vi "Do.vi"(8 "error in (no error)":errorcluster, 10 "Actor in":refnum<class "Actor.lvclass">, 11 "Mouseover Panel Object Msg":refnum<class "Mouseover Panel Object Msg.lvclass">) -> (0 "error out":errorcluster, 2 "Actor out":refnum<class "Actor.lvclass">)   [LabVIEW 2017, in "Pane Relief Main UI.lvlib" / "Mouseover Panel Object Msg.lvclass"]
doc: "This VI delivers the message to the actor by calling the appropriate method(s) on the actor."
uses:
  Mouseover Panel Object Msg.lvclass
  <vilib>/ActorFramework/Actor/Actor.lvclass
  Pane Relief Main UI/Pane Relief Main UI.lvclass
  C:/Program Files (x86)/National Instruments/LabVIEW 2017/vi.lib/ActorFramework/Actor/Actor.lvclass
  Mouseover Panel Object Msg.lvclass/Mouseover Panel Object Msg.ctl
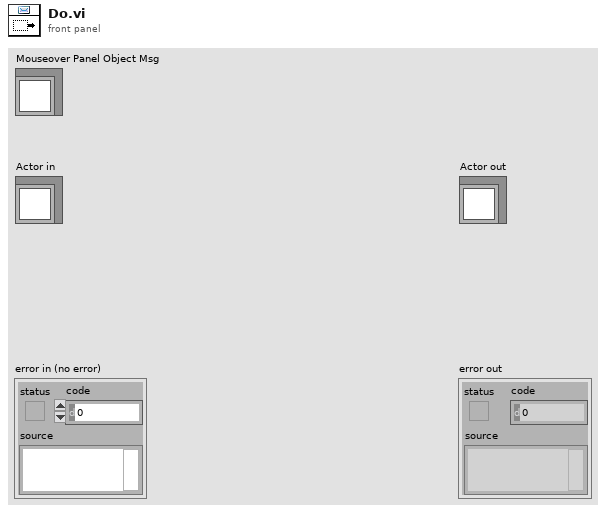
[diagram p1: front panel]
types:
  T1 = typedef "LVPoint32TypeDef.ctl" = cluster{"Horizontal":i32, "Vertical":i32}
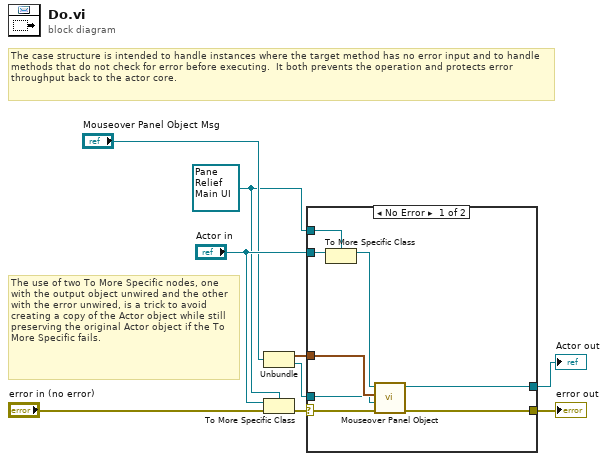
[diagram p0: block diagram]
diagram:
  w4 = refnum<class "Pane Relief Main UI.lvclass"> refnum ("Actor in")
  # "The use of two To More Specific nodes, one with the output object unwired and the other with the error unwired, is a trick to avoid creating a copy of the Actor object while still preserving the original Actor object if the To More Specific fails."
  # "The case structure is intended to handle instances where the target method has no error input and to handle methods that do not check for error before executing.  It both prevents the operation and protects error throughput back to the actor core."
  n1 = Unbundle("Mouseover Panel Object Msg") -> (w2:T1, w1:refnum<k4>)
  n2 = To More Specific Class(target class=w4, reference="Actor in", error in="error in (no error)") -> (error out=w3:errorcluster)  [unwired: 1 out]
  n3 = case shown="No Error" w3 {
    selector: w3 -> [w15 w19]
    tunnel: [w17 w19] -> w9
    tunnel: [w16 w18] -> w8
    tunnel: "Actor in" -> [w14 w18]
    tunnel: w4 -> [w13 _]
    tunnel: w2 -> [w11 _]
    tunnel: w1 -> [w10 _]
    frame No Error {
      n4 = To More Specific Class(target class=w13, reference=w14) -> (specific class reference=w12:refnum<class "Pane Relief Main UI.lvclass">)  [unwired: 1 in, 1 out]
      n5 = call-dynamic "Mouseover Panel Object.vi"("Error In"=w15, "Occurrence"=w10, "Coords"=w11, "Pane Relief Main UI in"=w12) -> ("Error Out"=w17:errorcluster, "Pane Relief Main UI out"=w16:refnum<class "Pane Relief Main UI.lvclass">)  [unwired: 6 in]
    }
    frame Error {
      # "If type check fails, pass the original object out again."
    }
  }
  "error out" <- w9
  "Actor out" <- w8
